vi "Init Msg.vi"(10 "Msg Input":refnum<class "Msg Input.lvclass">) -> (2 "Msg":refnum<class "Msg.lvclass">)   [LabVIEW 2020, in "jettl.lvlib" / "Start jettl Msg.lvlib" / "Start Msg.lvlib"]
doc: "jettl 6.14.1.98\nNathan Davis - Nathan Davis\nCopyright (c) 2026, Nathan Davis\nMIT"
uses:
  Start Msg.lvlib
  Msg/Msg.lvclass
  Msg Input/Msg Input.lvclass
  Start Msg/Start Msg.lvclass
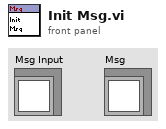
[diagram p1: front panel]
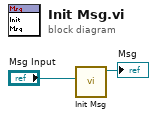
[diagram p0: block diagram]
diagram:
  n1 = call "Init Msg.vi"("Msg Input"="Msg Input") -> ("Start Msg out"=→"Msg":refnum<class "Start Msg.lvclass">)  [unwired: 10 in]
